vi "SDCP - Decode Standard Message Frame Parameter.vi"(2 "error in (no error)":errorcluster, 3 "Bytes in":u8[](array[numeric])) -> (0 "error out":errorcluster, 1 "SMF Parameters out":T1[](array[typedef]))   [LabVIEW 2020]
uses:
  Typedefs/SDCP - SMF parameter descriptors.ctl
  Typedefs/SDCP - Standard Message Frame Parameters - FGV - commands.ctl
  Typedefs/SDCP - Standard Message Frames FGV - Commands.ctl
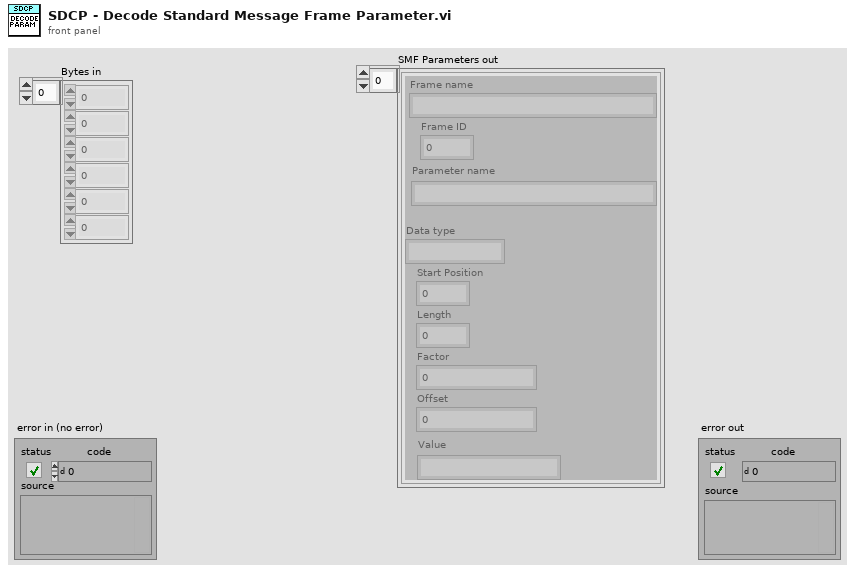
[diagram p1: front panel]
types:
  T1 = typedef "SDCP - SMF parameter descriptors.ctl" = cluster{"Frame name":string, "Frame ID":i32, "Data type":string, "Start Position":i32, "Length":i32, "Factor":dbl, "Offset":dbl, "Parameter name":string, "Value":string}
  T2 = typedef "SDCP - Standard Message Frame Parameters - FGV - commands.ctl" = enum16{"Write descriptors", "Read descriptors", "Read values", "Load parameters from file", "Write values", "Read all descriptors"}
  T3 = typedef "SDCP - Standard Message Frames FGV - Commands.ctl" = enum16{"Reset", "Read", "Write", "Set Priority"}
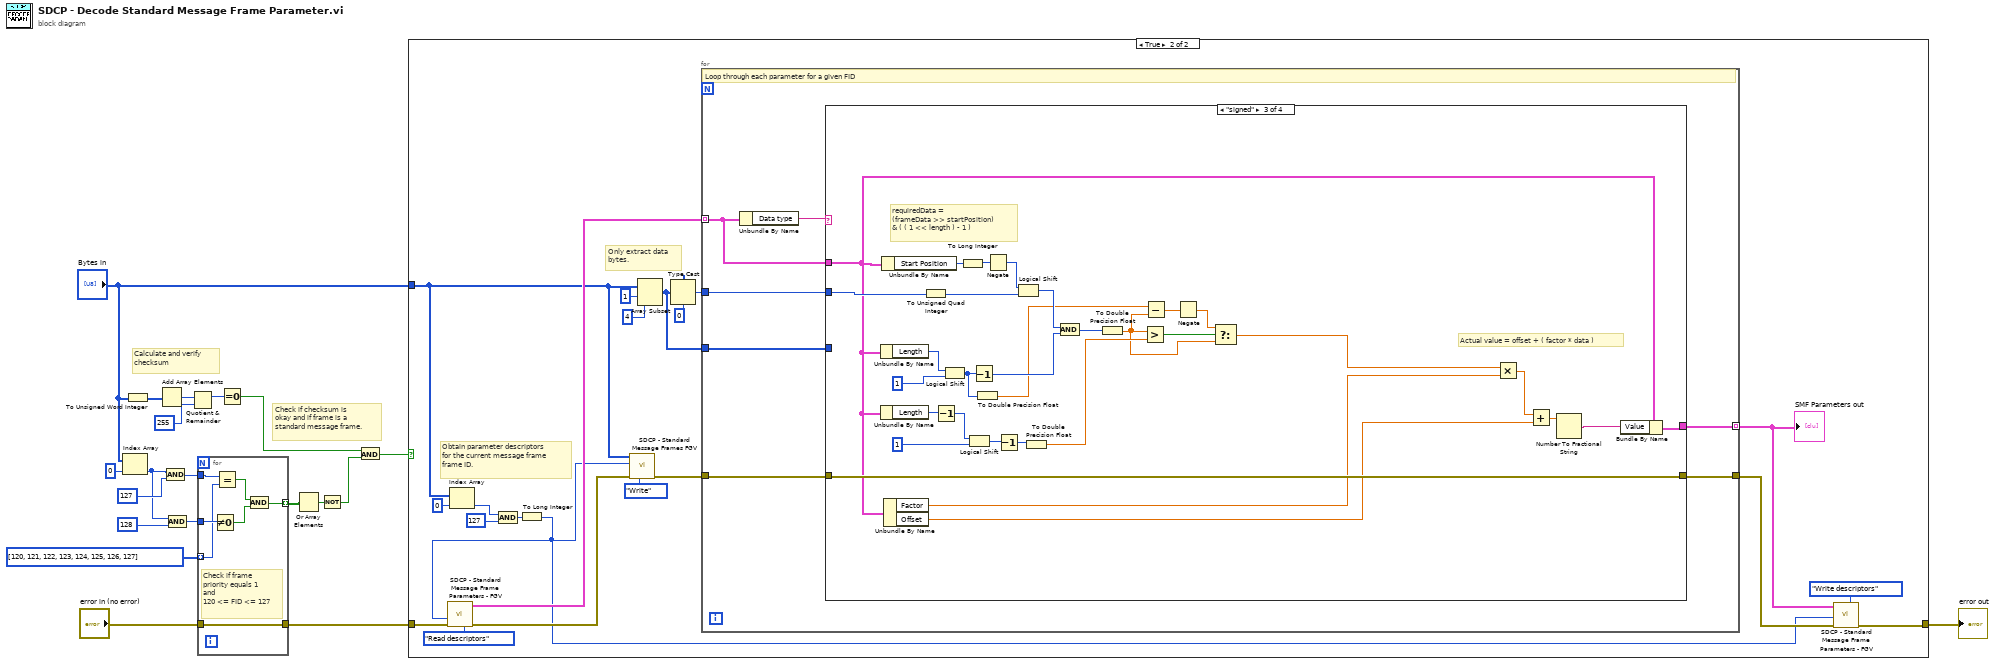
[diagram p0: block diagram]
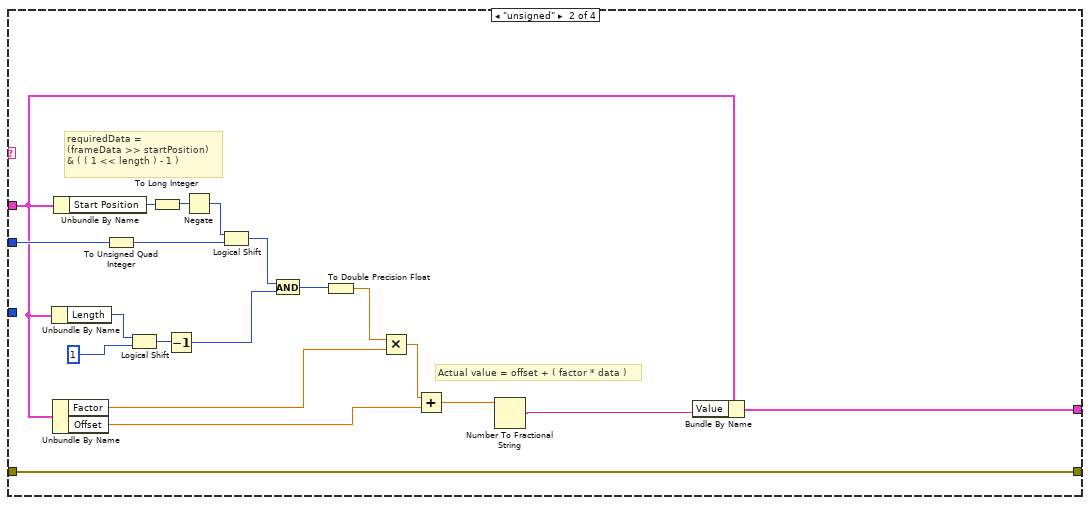
[diagram p4: hidden frame]
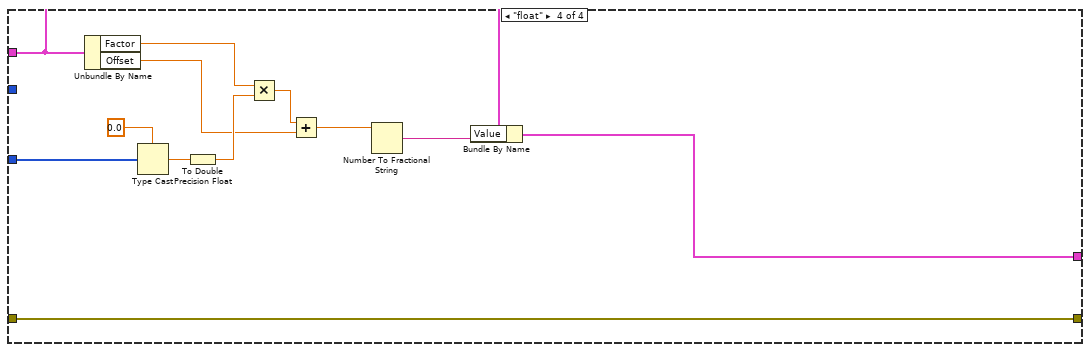
[diagram p5: hidden frame]
diagram:
  # "Check if checksum is\nokay and if frame is a\nstandard message frame."
  # "Calculate and verify\nchecksum"
  n1 = Index Array(array="Bytes in", index=0) -> (element=w13:u8)
  n2 = To Unsigned Word Integer(number="Bytes in") -> (unsigned 16bit integer=w20:u16[])
  n3 = Add Array Elements(numeric array=w20) -> (sum=w19:u16)
  n4 = And(x=w13, y=u8 127) -> (x .and. y?=w7:u8)
  n5 = And(x=w13, y=u8 128) -> (x .and. y?=w8:u8)
  n6 = Quotient & Remainder(x=w19, y=u16 255) -> (x-y*floor(x/y)=w17:u16)  [unwired: 1 out]
  n7 = for {
    tunnel: "error in (no error)" -> [w27]
    tunnel: [w27] -> w10
    tunnel: u8[] [120, 121, 122, 123, 124, 125, 126, 127] -> [w24] mode=indexing
    tunnel: w8 -> [w26]
    tunnel: w7 -> [w25]
    tunnel: [w21] -> w6 mode=indexing
    # "Check if frame\npriority equals 1\nand \n120 <= FID <= 127"
    n8 = Not Equal To 0?(x=w26) -> (x != 0?=w22:bool)
    n9 = Equal?(x=w25, y=w24) -> (x = y?=w23:bool)
    n10 = And(x=w23, y=w22) -> (x .and. y?=w21:bool)
  }
  n11 = Equal To 0?(x=w17) -> (x = 0?=w3:bool)
  n12 = Or Array Elements(Boolean array=w6) -> (logical OR=w5:bool)
  n13 = Not(x=w5) -> (.not. x?=w4:bool)
  n14 = And(x=w3, y=w4) -> (x .and. y?=w2:bool)
  n15 = case shown="True" w2 {
    tunnel: w10 -> [w28 w46]
    tunnel: [w28 w32] -> w16
    tunnel: "Bytes in" -> [_ w39]
    frame False {
    }
    frame True {
      # "Only extract data\nbytes."
      # "Obtain parameter descriptors\nfor the current message frame\nframe ID."
      n16 = Index Array(array=w39, index=0) -> (element=w48:u8)
      n17 = And(x=w48, y=u8 127) -> (x .and. y?=w45:u8)
      n18 = To Long Integer(number=w45) -> (32bit integer=w29:i32)
      n19 = call "SDCP - Standard Message Frame Parameters - FGV.vi"("FID"=w29, "error in (no error)"=w46, "Command"=SDCP_-_Standard_Message_Frame_Parameters_-_FGV_-_commands."Read descriptors") -> ("SMF Parameters descriptors out"=w43:T1[], "error out"=w42:errorcluster)  [unwired: 4 in]
      n20 = call "SDCP - Standard Message Frames FGV.vi"("error in (no error)"=w42, "Command"=SDCP_-_Standard_Message_Frames_FGV_-_Commands."Write", "FID"=w29, "SMF in"=w39) -> ("error out"=w41:errorcluster)  [unwired: 2 in, 2 out]
      n21 = Array Subset(array=w39, index=1, length=4) -> (w34:u8[])
      n22 = Type Cast(type=u32 0, x=w34) -> (*(type *) &x=w35:u32)
      n23 = for {
        tunnel: w43 -> [w55] mode=indexing
        tunnel: w41 -> [w53]
        tunnel: w35 -> [w54]
        tunnel: [w52] -> w33
        tunnel: [w51] -> w31 mode=indexing
        tunnel: w34 -> [w50]
        # "Loop through each parameter for a given FID"
        n24 = Unbundle By Name(w55) -> ("Data type"=w56:string)
        n25 = case shown="\"signed\"" w56 {
          tunnel: w55 -> [w57 w62 w92 w112]
          tunnel: w54 -> [_ w75 w97 _]
          tunnel: w53 -> [w58 w59 w96 w114]
          tunnel: [w58 w59 w96 w114] -> w52
          tunnel: [w57 w60 w95 w110] -> w51
          tunnel: w50 -> [_ _ _ w121]
          frame Default {
          }
          frame "unsigned" {
            # "Actual value = offset + ( factor * data )"
            # "requiredData = \n(frameData >> startPosition) \n& ( ( 1 << length ) - 1 )"
            n26 = Unbundle By Name(w62) -> ("Length"=w78:i32)
            n27 = Unbundle By Name(w62) -> ("Factor"=w66:dbl, "Offset"=w64:dbl)
            n28 = Unbundle By Name(w62) -> ("Start Position"=w74:i32)
            n29 = To Unsigned Quad Integer(1:w75) -> (0:w69:u64)
            n30 = Logical Shift(y=w78, x=u64 1) -> (x << y=w76:u64)
            n31 = To Long Integer(number=w74) -> (32bit integer=w73:i32)
            n32 = Decrement(x=w76) -> (x-1=w70:u64)
            n33 = Negate(x=w73) -> (-x=w72:i32)
            n34 = Logical Shift(y=w72, x=w69) -> (x << y=w71:u64)
            n35 = And(x=w71, y=w70) -> (x .and. y?=w68:u64)
            n36 = To Double Precision Float(number=w68) -> (double precision float=w67:dbl)
            n37 = Multiply(x=w67, y=w66) -> (x*y=w65:dbl)
            n38 = Add(x=w65, y=w64) -> (x+y=w63:dbl)
            n39 = Number To Fractional String(number=w63) -> (F-format string=w61:string)  [unwired: 3 in]
            n40 = Bundle By Name(cluster=w62, "Value"=w61) -> (w60:T1)
          }
          frame "signed" {
            # "Actual value = offset + ( factor * data )"
            # "requiredData = \n(frameData >> startPosition) \n& ( ( 1 << length ) - 1 )"
            n41 = Unbundle By Name(w92) -> ("Length"=w109:i32)
            n42 = Unbundle By Name(w92) -> ("Length"=w91:i32)
            n43 = Unbundle By Name(w92) -> ("Start Position"=w107:i32)
            n44 = Unbundle By Name(w92) -> ("Factor"=w81:dbl, "Offset"=w80:dbl)
            n45 = To Unsigned Quad Integer(1:w97) -> (0:w102:u64)
            n46 = Decrement(x=w91) -> (x-1=w90:i32)
            n47 = Logical Shift(y=w109, x=u64 1) -> (x << y=w86:u64)
            n48 = To Long Integer(number=w107) -> (32bit integer=w106:i32)
            n49 = Logical Shift(y=w90, x=u64 1) -> (x << y=w93:u64)
            n50 = Decrement(x=w86) -> (x-1=w103:u64)
            n51 = To Double Precision Float(number=w86) -> (double precision float=w85:dbl)
            n52 = Negate(x=w106) -> (-x=w105:i32)
            n53 = Decrement(x=w93) -> (x-1=w89:u64)
            n54 = Logical Shift(y=w105, x=w102) -> (x << y=w104:u64)
            n55 = To Double Precision Float(number=w89) -> (double precision float=w88:dbl)
            n56 = And(x=w104, y=w103) -> (x .and. y?=w101:u64)
            n57 = To Double Precision Float(number=w101) -> (double precision float=w83:dbl)
            n58 = Greater?(x=w83, y=w88) -> (0:w87:bool)
            n59 = Subtract(x=w85, y=w83) -> (x-y=w84:dbl)
            n60 = Negate(x=w84) -> (-x=w79:dbl)
            n61 = Select(t=w79, s=w87, f=w83) -> (s? t:f=w82:dbl)
            n62 = Multiply(x=w82, y=w81) -> (x*y=w100:dbl)
            n63 = Add(x=w100, y=w80) -> (x+y=w99:dbl)
            n64 = Number To Fractional String(number=w99) -> (F-format string=w98:string)  [unwired: 3 in]
            n65 = Bundle By Name(cluster=w92, "Value"=w98) -> (w95:T1)
          }
          frame "float" {
            n66 = Unbundle By Name(w112) -> ("Factor"=w118:dbl, "Offset"=w115:dbl)
            n67 = Type Cast(type=sgl 0.0 ("number"), x=w121) -> (*(type *) &x=w119:sgl)
            n68 = To Double Precision Float(number=w119) -> (double precision float=w117:dbl)
            n69 = Multiply(x=w118, y=w117) -> (x*y=w116:dbl)
            n70 = Add(x=w116, y=w115) -> (x+y=w113:dbl)
            n71 = Number To Fractional String(number=w113) -> (F-format string=w111:string)  [unwired: 3 in]
            n72 = Bundle By Name(cluster=w112, "Value"=w111) -> (w110:T1)
          }
        }
      }
      "SMF Parameters out" <- w31
      n73 = call "SDCP - Standard Message Frame Parameters - FGV.vi"("SMF Parameters descriptors in"=w31, "FID"=w29, "error in (no error)"=w33, "Command"=SDCP_-_Standard_Message_Frame_Parameters_-_FGV_-_commands."Write descriptors") -> ("error out"=w32:errorcluster)  [unwired: 3 in, 1 out]
    }
  }
  "error out" <- w16
